vi "Simulator VNA Config Test.vi"(4 "error in (no error)":errorcluster, 6 "Configuration":T1={"BusType"=enum."GPIB", "GPIB Bus"=0, "GPIB Address"=16, "IP"=0, "COM"=1, "Baud Rate"=enum."9600", "USB Device"=0, "Instrument S\\N"="", "SCIL Address"=16} {"USB Device" max=31 step=1}, 7 "Str Refnum":refnum<vi>) -> (0 "error out":errorcluster)   [LabVIEW 2011]
uses:
  VNA Configuration.ctl
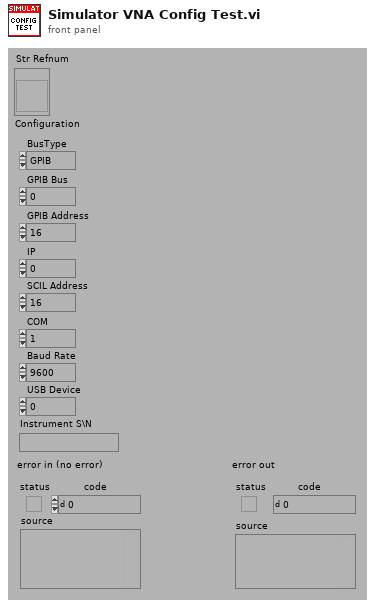
[diagram p1: front panel]
types:
  T1 = typedef "VNA Configuration.ctl" = cluster{"BusType":enum32{"GPIB", "LAN/IP", "Serial", "USB"}, "GPIB Bus":i32, "GPIB Address":i32, "IP":u32, "COM":i32, "Baud Rate":enum32{"300", "600", "1200", "2400", "4800", "9600"}, "USB Device":u32, "Instrument S\\N":string, "SCIL Address":i32}
  T2 = enum32{"300", "600", "1200", "2400", "4800", "9600"}
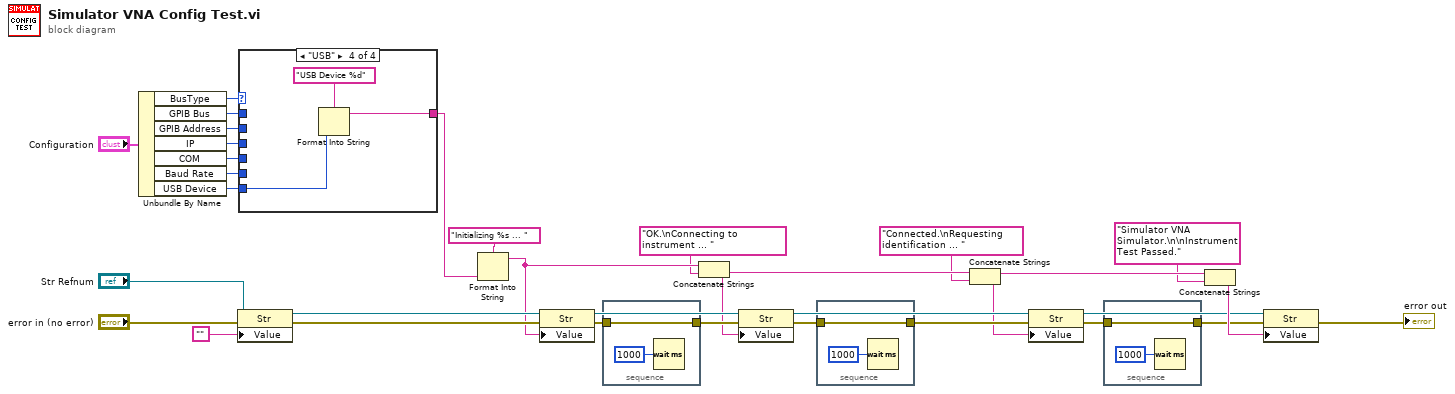
[diagram p0: block diagram]
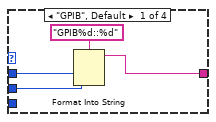
[diagram p2: hidden frame]
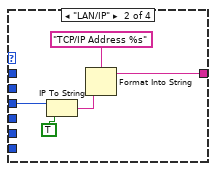
[diagram p3: hidden frame]
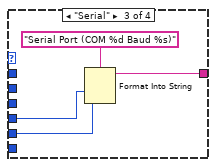
[diagram p4: hidden frame]
diagram:
  n1 = Unbundle By Name("Configuration") -> ("BusType"=w26:enum32{"GPIB", "LAN/IP", "Serial", "USB"}, "GPIB Bus"=w25:i32, "GPIB Address"=w24:i32, "IP"=w23:u32, "COM"=w22:i32, "Baud Rate"=w2:T2, "USB Device"=w1:u32)
  n2 = property class="Str"(reference="Str Refnum", error in="error in (no error)", "Value"="") -> (reference out=w19:refnum<vi>, error out=w29:errorcluster)
  n3 = case shown="\"USB\"" w26 {
    tunnel: w25 -> [w35 _ _ _]
    tunnel: w24 -> [w34 _ _ _]
    tunnel: w23 -> [_ w40 _ _]
    tunnel: w22 -> [_ _ w44 _]
    tunnel: [w33 w37 w43 w47] -> w21
    tunnel: w2 -> [_ _ w42 _]
    tunnel: w1 -> [_ _ _ w46]
    frame "GPIB", Default {
      n4 = Format Into String(format string="GPIB%d::%d", w35, w34) -> (resulting string=w33:string)  [unwired: 2 in, 1 out]
    }
    frame "LAN/IP" {
      n5 = IP To String(1:TRUE, 2:w40) -> (0:w39:string)
      n6 = Format Into String(format string="TCP/IP Address %s", w39) -> (resulting string=w37:string)  [unwired: 2 in, 1 out]
    }
    frame "Serial" {
      n7 = Format Into String(format string="Serial Port (COM %d Baud %s)", w44, w42) -> (resulting string=w43:string)  [unwired: 2 in, 1 out]
    }
    frame "USB" {
      n8 = Format Into String(format string="USB Device %d", w46) -> (resulting string=w47:string)  [unwired: 2 in, 1 out]
    }
  }
  n9 = Format Into String(format string="Initializing %s ... ", w21) -> (resulting string=w12:string)  [unwired: 2 in, 1 out]
  n10 = property class="Str"(reference=w19, error in=w29, "Value"=w12) -> (reference out=w17:refnum<vi>, error out=w20:errorcluster)
  n11 = stacked-sequence {
    tunnel: w20 -> [w49]
    tunnel: [w49] -> w18
    frame #0 {
      n12 = Wait (ms)(milliseconds to wait=u32 1000) -> ()  [unwired: 1 out]
    }
  }
  n13 = Concatenate Strings(w12, "OK.\nConnecting to instrument ... ") -> (w10:string)
  n14 = property class="Str"(reference=w17, error in=w18, "Value"=w10) -> (reference out=w14:refnum<vi>, error out=w16:errorcluster)
  n15 = stacked-sequence {
    tunnel: w16 -> [w51]
    tunnel: [w51] -> w15
    frame #0 {
      n16 = Wait (ms)(milliseconds to wait=u32 1000) -> ()  [unwired: 1 out]
    }
  }
  n17 = Concatenate Strings(w10, "Connected.\nRequesting identification ... ") -> (w6:string)
  n18 = property class="Str"(reference=w14, error in=w15, "Value"=w6) -> (reference out=w3:refnum<vi>, error out=w13:errorcluster)
  n19 = stacked-sequence {
    tunnel: w13 -> [w53]
    tunnel: [w53] -> w7
    frame #0 {
      n20 = Wait (ms)(milliseconds to wait=u32 1000) -> ()  [unwired: 1 out]
    }
  }
  n21 = Concatenate Strings(w6, "Simulator VNA Simulator.\n\nInstrument Test Passed.") -> (w8:string)
  n22 = property class="Str"(reference=w3, error in=w7, "Value"=w8) -> (error out=→"error out":errorcluster)  [unwired: 1 out]
